vi "set_indexArray.vi"(0 "HGF_FGV_VisitSelection":refnum<class "HGF_FGV_VisitSelection.lvclass">, 2 "indexArray":u32[](array[numeric]), 5 "error in (no error)":errorcluster) -> (14 "dup HGF_FGV_VisitSelection":refnum<class "HGF_FGV_VisitSelection.lvclass">, 19 "error out":errorcluster)   [LabVIEW 2012, in "HGF_FGV.lvlib" / "HGF_FGV_VisitSelection.lvclass"]
doc: "Set index array."
uses:
  HGF_FGV_VisitSelection.lvclass
  HGF_FGV_VisitSelection.lvclass/HGF_FGV_VisitSelection.ctl
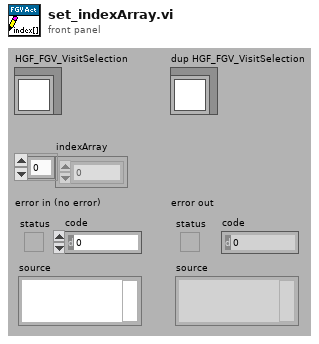
[diagram p1: front panel]
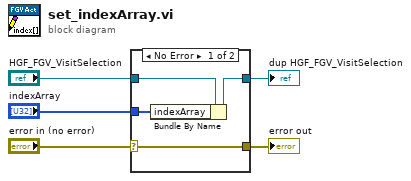
[diagram p0: block diagram]
diagram:
  n1 = case shown="No Error" "error in (no error)" {
    selector: "error in (no error)" -> [w9 w10]
    tunnel: [w9 w10] -> w4
    tunnel: [w7 w11] -> w2
    tunnel: "HGF_FGV_VisitSelection" -> [w8 w11]
    tunnel: "indexArray" -> [w6 _]
    frame No Error {
      n2 = Bundle By Name(cluster=w8, "indexArray"=w6) -> (w7:refnum<class "HGF_FGV_VisitSelection.lvclass">)
    }
    frame Error {
    }
  }
  "error out" <- w4
  "dup HGF_FGV_VisitSelection" <- w2
